vi "robust_set_cursor.vi"   [LabVIEW 2015]
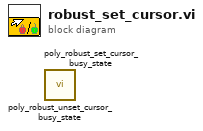
[diagram p0: block diagram]
diagram:
  n1 = call "poly_robust_unset_cursor_busy_state.vi"() -> ()  [unwired: 10 in, 2 out]
  n2 = call "poly_robust_set_cursor_busy_state.vi"() -> ()  [unwired: 10 in, 2 out]
